vi "unhandled message received.vi"(9 "unhandledMessage":string, 11 "queues":T1) -> ()   [LabVIEW 2018]
uses:
  type defs/Queues.ctl
  <vilib>/ErrorRing/Error Ring.xnode
panel:
  out "error out":errorcluster
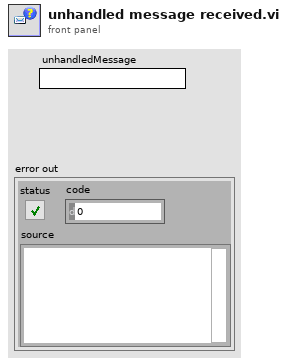
[diagram p1: front panel]
types:
  T1 = typedef "Queues.ctl" = cluster{"messageHandler":refnum<queue>, "comms":refnum<queue>, "dataStream":refnum<queue>, "dataProcessor":refnum<queue>, "fileIO":refnum<queue>, "userInterface":refnum<queue>, "errors":refnum<queue>, "customCompressor":refnum<queue>}
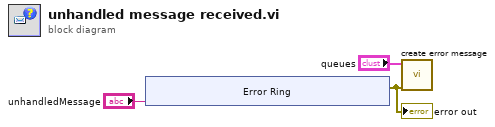
[diagram p0: block diagram]
diagram:
  n1 = xnode "Error Ring"("parameter 0"="unhandledMessage") -> ("error out"=w3:errorcluster)
  "error out" <- w3
  n2 = call "create error message.vi"("error in (no error)"=w3, "queues"="queues") -> ()  [unwired: 10 in]
